vi "Test_IronPythonSaves.vi"() -> ()   [LabVIEW 2014]
uses:
  Hardware Control/Spectrometer/Spectral Data.ctl
  Hardware Control/Parameter Analyzer/Electrical Data.ctl
  SaveData Function.ctl
  SaveData Instrument Configuration.ctl
  Instrument Sequence/Instrument List.ctl
panel:
  in  "Electrical Measurement Data":T1={"Sequence"=[0.0], "V1"=[0.0, 1.0, 2.0], "V2"=[0.0, 1.0, 2.0], "V3"=[0.0, 1.0, 2.0], "V4"=[0.0, 1.0, 2.0], "I1"=[0.0, -1.0, -2.0], "I2"=[0.0, -1.0, -2.0], "I3"=[0.0, -1.0, -2.0], "I4"=[0.0, -1.0, -2.0]}
  out "output cluster":T2={"Intensity"=[2.0, 0.0, -2.0], "Wavelength"=[2.0, 0.0, -2.0], "Energy"=[2.0, 0.0, -2.0], "Raman Shift"=[2.0, 0.0, -2.0], "Detector Temperature"=0.0}
  in  "Save Data":T3={"Device Name"="test", "Device Info"="test", "Path"=path "C:/Users/gio/Desktop/test python/test.pmat"}
  out "error out":errorcluster
  # "LICENSED MATERIALS – PROPERTY OF IBM\nCopyright IBM Corp. 2016,\nALL RIGHTS RESERVED"
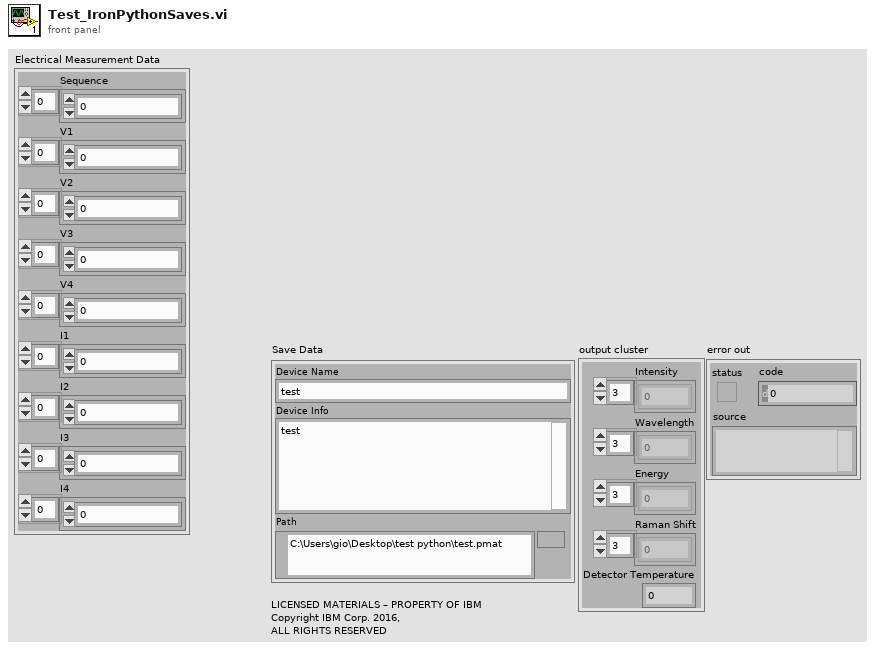
[diagram p1: front panel]
types:
  T1 = typedef "Electrical Data.ctl" = cluster{"Sequence":dbl[], "V1":dbl[], "V2":dbl[], "V3":dbl[], "V4":dbl[], "I1":dbl[], "I2":dbl[], "I3":dbl[], "I4":dbl[]}
  T2 = typedef "Spectral Data.ctl" = cluster{"Intensity":dbl[], "Wavelength":dbl[], "Energy":dbl[], "Raman Shift":dbl[], "Detector Temperature":dbl}
  T3 = cluster{"Device Name":string, "Device Info":string, "Path":path}
  T4 = typedef "SaveData Function.ctl" = enum16{"Start Python Session", "Set Data Structures to Default", "Append Stress Data", "Append Electrical Measurement", "Append Optical Spectrum", "Append Stress Measurement Step", "Append Instrument Sequence Step", "Set Instrument Configuration", "Set Stress Data", "Set Electrical Measurement", "Set Optical Spectum", "Save Electrical Measurement", "Save Optical Spectrum", "Save Optoelectronic Measurement", "Save Instrument Sequence", "Save Stress Measurement", "Pickle2Workspace", "Explore Variable Space", "Close"}
  T5 = typedef "Instrument List.ctl" = enum32{"Unknown Instrument", "Switching Matrix", "Parameter Analyzer", "Optical Spectrometer", "Optoelectronic", "Autofocus"}
  T6 = typedef "SaveData Instrument Configuration.ctl" = cluster{"Instrument":T5, "Configuration":string}
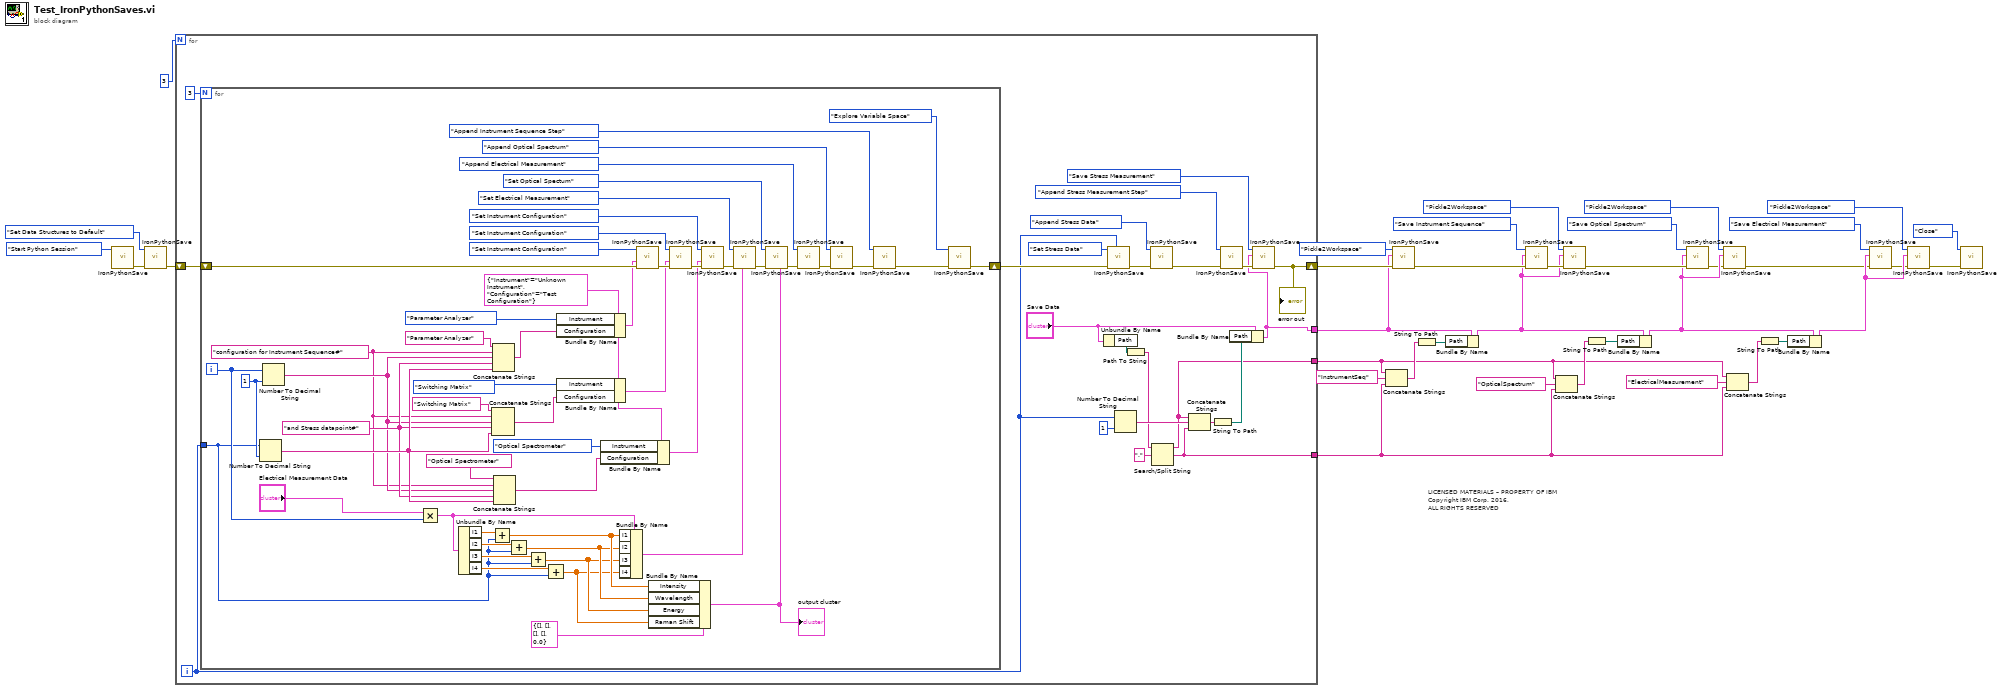
[diagram p0: block diagram]
diagram:
  # "LICENSED MATERIALS – PROPERTY OF IBM\nCopyright IBM Corp. 2016,\nALL RIGHTS RESERVED"
  n1 = call "IronPythonSave.vi"("Function"=SaveData_Function."Start Python Session") -> ("error out"=w33:errorcluster)  [unwired: 10 in]
  n2 = call "IronPythonSave.vi"("error in (no error)"=w33, "Function"=SaveData_Function."Set Data Structures to Default") -> ("error out"=w31:errorcluster)  [unwired: 9 in]
  n3 = for {
    N: 3 -> [_]
    shift-right: [w59] -> w29
    shift-left: w31 -> [w53]
    tunnel: [w39] -> w18
    tunnel: [w38] -> w2
    tunnel: [w37] -> w1
    i -> [w49]
    n4 = for {
      N: 3 -> [_]
      shift-right: [w64] -> w54
      shift-left: w53 -> [w102]
      tunnel: w49 -> [w94]
      i -> [w100]
      w82 = T6 {"Instrument"=enum."Unknown Instrument", "Configuration"="Test Configuration"} ("Instrument Configuration")
      w101 = i16 1 ("width (-)")
      w85 = "and Stress datapoint#" ("Configuration")
      w83 = "configuration for Instrument Sequence#" ("Configuration")
      n5 = Number To Decimal String(number=w94, width (-)=w101) -> (decimal integer string=w86:string)
      n6 = Number To Decimal String(number=w100, width (-)=w101) -> (decimal integer string=w84:string)
      n7 = Multiply(x="Electrical Measurement Data", y=w100) -> (x*y=w99:T1)
      n8 = Unbundle By Name(w99) -> ("I1"=w95:dbl[], "I2"=w96:dbl[], "I3"=w97:dbl[], "I4"=w98:dbl[])
      n9 = Add(x=w95, y=w94) -> (x+y=w69:dbl[])
      n10 = Concatenate Strings("Switching Matrix" ("Configuration"), w83, w84, w85, w86) -> (w104:string)
      n11 = Concatenate Strings("Parameter Analyzer" ("Configuration"), w83, w84, w85, w86) -> (w105:string)
      n12 = Concatenate Strings("Optical Spectrometer" ("Configuration"), w83, w84, w85, w86) -> (w78:string)
      n13 = Add(x=w96, y=w94) -> (x+y=w68:dbl[])
      n14 = Add(x=w97, y=w94) -> (x+y=w67:dbl[])
      n15 = Add(x=w98, y=w94) -> (x+y=w66:dbl[])
      n16 = Bundle By Name(cluster=w82, "Instrument"=Instrument_List."Parameter Analyzer", "Configuration"=w105) -> (w92:T6)
      n17 = Bundle By Name(cluster=w82, "Instrument"=Instrument_List."Switching Matrix", "Configuration"=w104) -> (w93:T6)
      n18 = Bundle By Name(cluster=w82, "Instrument"=Instrument_List."Optical Spectrometer", "Configuration"=w78) -> (w77:T6)
      n19 = Bundle By Name(cluster=w99, "I1"=w69, "I2"=w68, "I3"=w67, "I4"=w66) -> (w75:T1)
      n20 = call "IronPythonSave.vi"("error in (no error)"=w102, "Instrument Configuration"=w92, "Function"=SaveData_Function."Set Instrument Configuration") -> ("error out"=w110:errorcluster)  [unwired: 8 in]
      n21 = Bundle By Name(cluster=T2 {"Intensity"=[], "Wavelength"=[], "Energy"=[], "Raman Shift"=[], "Detector Temperature"=0.0} ("Optical Spectrum"), "Intensity"=w69, "Wavelength"=w68, "Energy"=w67, "Raman Shift"=w66) -> (w70:T2)
      "output cluster" <- w70
      n22 = call "IronPythonSave.vi"("error in (no error)"=w110, "Instrument Configuration"=w93, "Function"=SaveData_Function."Set Instrument Configuration") -> ("error out"=w89:errorcluster)  [unwired: 8 in]
      n23 = call "IronPythonSave.vi"("error in (no error)"=w89, "Instrument Configuration"=w77, "Function"=SaveData_Function."Set Instrument Configuration") -> ("error out"=w74:errorcluster)  [unwired: 8 in]
      n24 = call "IronPythonSave.vi"("Electrical Measurement"=w75, "error in (no error)"=w74, "Function"=SaveData_Function."Set Electrical Measurement") -> ("error out"=w61:errorcluster)  [unwired: 8 in]
      n25 = call "IronPythonSave.vi"("Optical Spectrum"=w70, "error in (no error)"=w61, "Function"=SaveData_Function."Set Optical Spectum") -> ("error out"=w62:errorcluster)  [unwired: 8 in]
      n26 = call "IronPythonSave.vi"("error in (no error)"=w62, "Function"=SaveData_Function."Append Electrical Measurement") -> ("error out"=w60:errorcluster)  [unwired: 9 in]
      n27 = call "IronPythonSave.vi"("error in (no error)"=w60, "Function"=SaveData_Function."Append Optical Spectrum") -> ("error out"=w91:errorcluster)  [unwired: 9 in]
      n28 = call "IronPythonSave.vi"("error in (no error)"=w91, "Function"=SaveData_Function."Append Instrument Sequence Step") -> ("error out"=w65:errorcluster)  [unwired: 9 in]
      n29 = call "IronPythonSave.vi"("error in (no error)"=w65, "Function"=SaveData_Function."Explore Variable Space") -> ("error out"=w64:errorcluster)  [unwired: 9 in]
    }
    n30 = Unbundle By Name("Save Data") -> ("Path"=w51:path)
    n31 = call "IronPythonSave.vi"("Stress Motor Position"=w49, "error in (no error)"=w54, "Function"=SaveData_Function."Set Stress Data") -> ("error out"=w44:errorcluster)  [unwired: 8 in]
    n32 = Number To Decimal String(number=w49, width (-)=i16 1) -> (decimal integer string=w48:string)
    n33 = Path To String(path=w51) -> (string=w41:string)
    n34 = call "IronPythonSave.vi"("error in (no error)"=w44, "Function"=SaveData_Function."Append Stress Data") -> ("error out"=w43:errorcluster)  [unwired: 9 in]
    n35 = Search/Split String(string=w41, search string/char (-)=".") -> (substring before match=w38:string, match + rest of string=w37:string)  [unwired: 2 out]
    n36 = Concatenate Strings(w38, w48, w37) -> (w46:string)
    n37 = String To Path(string=w46) -> (path=w45:path)
    n38 = call "IronPythonSave.vi"("error in (no error)"=w43, "Function"=SaveData_Function."Append Stress Measurement Step") -> ("error out"=w57:errorcluster)  [unwired: 9 in]
    n39 = Bundle By Name(cluster="Save Data", "Path"=w45) -> (w39:T3)
    n40 = call "IronPythonSave.vi"("error in (no error)"=w57, "Workspace Info"=w39, "Function"=SaveData_Function."Save Stress Measurement") -> ("error out"=w59:errorcluster)  [unwired: 8 in]
    "error out" <- w59
  }
  n41 = Concatenate Strings(w2, "InstrumentSeq" ("search string/char (-)"), w1) -> (w11:string)
  n42 = call "IronPythonSave.vi"("error in (no error)"=w29, "Workspace Info"=w18, "Function"=SaveData_Function."Pickle2Workspace") -> ("error out"=w27:errorcluster)  [unwired: 8 in]
  n43 = String To Path(string=w11) -> (path=w12:path)
  n44 = Bundle By Name(cluster=w18, "Path"=w12) -> (w17:T3)
  n45 = call "IronPythonSave.vi"("error in (no error)"=w27, "Workspace Info"=w17, "Function"=SaveData_Function."Save Instrument Sequence") -> ("error out"=w25:errorcluster)  [unwired: 8 in]
  n46 = Concatenate Strings(w2, "OpticalSpectrum" ("search string/char (-)"), w1) -> (w10:string)
  n47 = call "IronPythonSave.vi"("error in (no error)"=w25, "Workspace Info"=w17, "Function"=SaveData_Function."Pickle2Workspace") -> ("error out"=w20:errorcluster)  [unwired: 8 in]
  n48 = String To Path(string=w10) -> (path=w14:path)
  n49 = Bundle By Name(cluster=w17, "Path"=w14) -> (w16:T3)
  n50 = call "IronPythonSave.vi"("error in (no error)"=w20, "Workspace Info"=w16, "Function"=SaveData_Function."Save Optical Spectrum") -> ("error out"=w5:errorcluster)  [unwired: 8 in]
  n51 = call "IronPythonSave.vi"("error in (no error)"=w5, "Workspace Info"=w16, "Function"=SaveData_Function."Pickle2Workspace") -> ("error out"=w3:errorcluster)  [unwired: 8 in]
  n52 = Concatenate Strings(w2, "ElectricalMeasurement" ("search string/char (-)"), w1) -> (w9:string)
  n53 = String To Path(string=w9) -> (path=w13:path)
  n54 = Bundle By Name(cluster=w16, "Path"=w13) -> (w15:T3)
  n55 = call "IronPythonSave.vi"("error in (no error)"=w3, "Workspace Info"=w15, "Function"=SaveData_Function."Save Electrical Measurement") -> ("error out"=w4:errorcluster)  [unwired: 8 in]
  n56 = call "IronPythonSave.vi"("error in (no error)"=w4, "Workspace Info"=w15, "Function"=SaveData_Function."Pickle2Workspace") -> ("error out"=w19:errorcluster)  [unwired: 8 in]
  n57 = call "IronPythonSave.vi"("error in (no error)"=w19, "Function"=SaveData_Function."Close") -> ()  [unwired: 9 in, 1 out]
